vi "day 9 task 1.vi"() -> ()   [LabVIEW 2019]
uses:
  00c26ec4-7482-4959-871a-3b0b3985b684.vi
panel:
  out "Final T pos":cluster{"x":i32, "y":i32}
  out "Final H pos":cluster{"x":i32, "y":i32}
  out "size(s)":i32
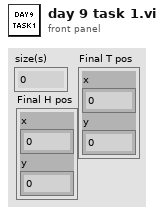
[diagram p1: front panel]
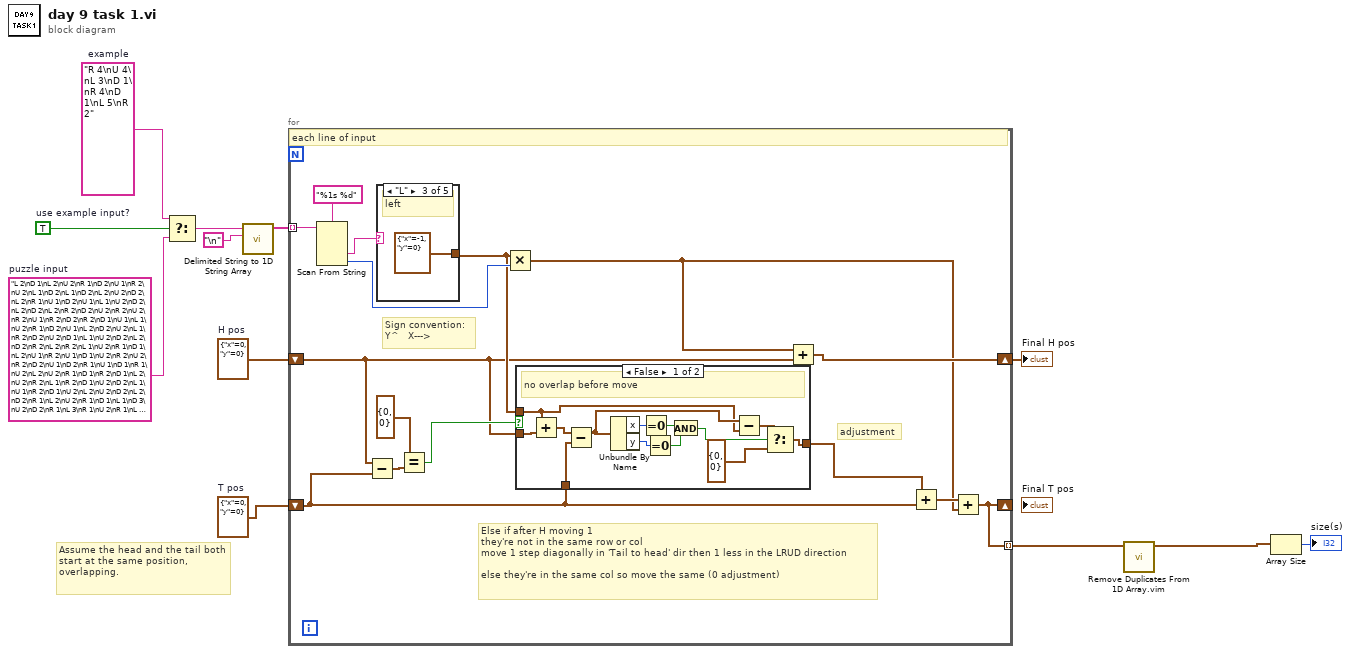
[diagram p0: block diagram]
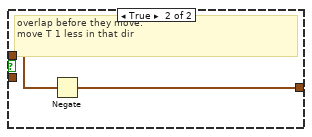
[diagram p2: hidden frame]
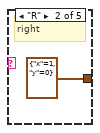
[diagram p4: hidden frame]
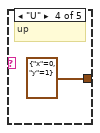
[diagram p5: hidden frame]
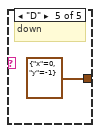
[diagram p6: hidden frame]
diagram:
  w5 = cluster{"x":i32, "y":i32} {"x"=0, "y"=0}  # T pos
  w6 = cluster{"x":i32, "y":i32} {"x"=0, "y"=0}  # H pos
  w10 = "R 4\nU 4\nL 3\nD 1\nR 4\nD 1\nL 5\nR 2"  # example
  w11 = TRUE  # use example input?
  w12 = "L 2\nD 1\nL 2\nU 2\nR 1\nD 2\nU 1\nR 2\nU 2\nL 1\nD 2\nL 1\nD 2\nL 2\nU 2\nD 2\nL 2\nR 1\nU 1\nD 2\nU 1\nL 1\nU 2\nD 2\nL 2\nD 2\nL 2\nR 2\nD 2\nU 2\nR 2\nU 2\nR 2\nU 1\nR 2\nD 2\nR 2\nD 1\nU 1\nL 1\nU 2\nR 1\nD 2\nU 1\nL 2\nD 2\nU 2\nL 1\nR 2\nD 2\nU 2\nD 1\nL 1\nU 2\nD 2\nL 2\nD 2\nR 2\nL 2\nR 2\nL 1\nU 2\nR 1\nD 1\nL 2\nU 1\nR 2\nU 1\nD 1\nU 2\nR 2\nU 2\nR 2\nD 2\nU 1\nD 2\nR 1\nU 1\nD 1\nR 1\nU 2\nL 2\nU 2\nR 1\nD 1\nR 2\nD 1\nL 2\nU 2\nR 2\nL 1\nR 2\nD 1\nU 2\nD 2\nL 1\nU 1\nR 2\nD 1\nU 2\nL 2\nU 2\nD 2\nL 2\nD 2\nR 1\nL 2\nU 2\nR 1\nD 1\nL 1\nD 3\nU 2\nD 2\nR 1\nL 3\nR 1\nU 2\nR 1\nL 2\nU 1\nL 3\nR 2\nU 2\nR 3\nU 3\nL 3\nU 1\nD 1\nR 3\nL 2\nU 1\nR 2\nU 1\nD 3\nU 1\nR 2\nL 2\nD 1\nL 1\nR 3\nU 2\nL 3\nR 2\nD 2\nL 1\nU 2\nR 2\nU 3\nL 1\nR 2\nL 3\nU 3\nL 1\nU 2\nR 2\nU 2\nD 2\nL 2\nU 1\nD 1\nU 2\nD 3\nR 2\nL 2\nU 1\nR 2\nD 3\nU 2\nL 2\nU 1\nR 1\nL 1\nD 1\nL 3\nR 2\nD 2\nL 2\nD 1\nU 3\nD 3\nU 3\nL 3\nR 2\nL 1\nU 2\nR 3\nU 2\nR 2\nU 3\nD 2\nU 1\nL 3\nU 1\nL 1\nD 2\nL 2\nR 1\nL 1\nD 3\nL 2\nD 2\nR 2\nL 3\nR 2\nL 2\nU 1\nL 3\nU 2\nR 2\nD 2\nU 2\nL 1\nD 3\nR 1\nU 3\nD 2\nU 3\nL 1\nD 2\nR 1\nU 3\nR 4\nL 1\nU 4\nR 2\nD 2\nU 3\nD 1\nL 1\nD 4\nL 3\nD 4\nL 3\nD 3\nU 4\nL 2\nD 1\nU 1\nR 4\nD 4\nL 2\nR 3\nU 3\nD 1\nL 3\nD 2\nL 4\nD 4\nR 3\nD 4\nU 4\nR 3\nL 4\nU 1\nL 1\nR 4\nD 2\nR 4\nU 3\nD 2\nR 4\nU 4\nD 1\nU 2\nD 3\nU 2\nL 3\nR 4\nL 1\nU 4\nD 3\nL 4\nR 2\nU 1\nR 1\nD 2\nL 2\nU 2\nL 3\nR 1\nL 2\nD 1\nR 3\nL 4\nU 2\nR 1\nU 1\nR 3\nL 3\nD 2\nU 2\nL 1\nR 1\nL 2\nD 2\nL 1\nR 2\nL 1\nU 1\nR 1\nL 4\nR 3\nU 4\nR 4\nL 2\nR 4\nL 1\nU 2\nR 3\nL 4\nU 1\nR 1\nD 1\nU 3\nL 1\nD 2\nU 2\nD 3\nR 4\nU 1\nR 3\nD 2\nU 1\nD 1\nU 4\nR 2\nD 4\nL 3\nR 4\nU 3\nD 4\nL 3\nU 2\nD 2\nL 4\nD 1\nL 2\nR 2\nU 3\nR 5\nL 3\nU 5\nL 4\nU 3\nD 1\nU 2\nD 5\nL 5\nD 3\nR 3\nD 3\nU 3\nD 5\nU 4\nD 5\nL 5\nR 2\nD 1\nR 5\nU 2\nL 2\nU 5\nL 1\nR 4\nU 5\nR 1\nD 5\nR 3\nU 1\nR 5\nD 5\nL 1\nD 4\nR 5\nL 1\nD 3\nU 2\nD 1\nU 1\nD 4\nL 5\nD 4\nR 1\nL 2\nU 3\nL 1\nU 3\nL 3\nU 4\nL 2\nR 4\nD 5\nU 1\nL 3\nU 5\nR 1\nD 4\nU 3\nL 5\nU 1\nL 3\nD 3\nR 4\nL 5\nU 1\nL 5\nU 2\nD 1\nR 2\nL 2\nD 4\nL 5\nD 2\nR 5\nL 4\nD 1\nR 5\nU 3\nR 2\nD 3\nL 1\nD 1\nL 4\nU 5\nL 2\nD 3\nR 5\nU 2\nL 1\nU 5\nD 4\nU 1\nR 2\nL 1\nU 2\nL 3\nD 1\nU 3\nL 1\nR 5\nU 3\nR 3\nU 2\nR 5\nL 5\nU 1\nL 5\nD 5\nR 1\nU 4\nL 6\nD 4\nU 2\nL 1\nU 5\nL 1\nR 6\nD 3\nU 5\nR 3\nU 5\nD 3\nR 3\nL 2\nU 2\nL 6\nR 3\nU 5\nD 5\nL 6\nR 1\nL 1\nD 5\nU 1\nR 5\nL 4\nR 1\nL 5\nD 1\nL 2\nU 4\nL 5\nU 4\nR 2\nL 1\nD 2\nR 4\nU 5\nD 4\nU 2\nL 3\nR 2\nL 1\nD 3\nU 1\nL 2\nU 6\nL 2\nU 3\nR 2\nD 1\nL 4\nR 5\nL 3\nU 5\nL 6\nR 3\nU 4\nL 2\nR 3\nU 3\nL 1\nD 5\nR 5\nD 5\nU 5\nL 6\nR 5\nL 4\nU 2\nR 5\nU 1\nD 2\nR 2\nD 1\nU 6\nL 5\nD 1\nR 6\nU 5\nR 3\nD 1\nR 4\nD 2\nU 5\nL 5\nR 2\nD 2\nR 1\nU 4\nR 3\nU 4\nL 6\nD 3\nR 4\nL 4\nU 5\nD 1\nU 1\nD 5\nU 4\nL 5\nD 1\nR 1\nU 5\nD 7\nR 5\nD 2\nR 2\nD 7\nL 1\nR 2\nD 2\nR 7\nU 4\nD 3\nU 3\nD 3\nL 4\nD 2\nR 6\nL 7\nD 6\nU 4\nD 1\nL 4\nU 3\nD 1\nU 1\nL 6\nD 4\nL 7\nU 6\nR 4\nL 7\nU 2\nD 5\nL 7\nU 3\nR 3\nU 6\nR 7\nU 4\nR 4\nL 4\nU 6\nR 6\nD 7\nU 4\nD 5\nL 4\nU 7\nR 7\nD 3\nL 5\nU 7\nD 3\nU 1\nD 7\nR 7\nL 4\nU 7\nD 1\nR 3\nD 3\nU 4\nR 2\nU 4\nR 4\nU 7\nR 4\nL 2\nU 4\nR 7\nL 6\nU 1\nD 2\nU 3\nD 1\nL 6\nD 5\nL 7\nR 6\nD 6\nL 4\nD 4\nU 3\nD 3\nL 7\nR 7\nL 7\nD 6\nU 5\nD 7\nU 7\nD 4\nU 7\nL 6\nU 3\nD 3\nR 3\nD 4\nL 2\nU 2\nR 4\nD 5\nR 7\nU 7\nL 2\nU 1\nD 4\nU 3\nL 4\nU 6\nD 4\nL 4\nU 6\nD 5\nL 1\nR 4\nL 2\nD 6\nR 4\nD 3\nR 3\nL 1\nD 2\nU 3\nL 1\nU 7\nL 3\nR 5\nU 1\nL 4\nD 8\nL 7\nD 8\nL 4\nU 6\nR 2\nD 4\nR 3\nD 3\nR 6\nL 8\nR 6\nD 4\nL 5\nR 5\nD 3\nU 6\nD 5\nU 3\nL 1\nD 4\nU 2\nR 5\nD 8\nL 3\nD 2\nU 8\nL 2\nD 6\nL 6\nD 2\nR 8\nL 3\nD 8\nU 5\nL 1\nR 1\nD 3\nL 5\nR 7\nU 4\nD 1\nL 2\nD 2\nL 5\nD 7\nR 7\nU 5\nL 5\nD 6\nL 1\nU 3\nL 4\nR 6\nD 7\nU 1\nR 1\nL 8\nU 3\nD 4\nR 2\nD 8\nL 1\nR 8\nU 7\nL 6\nU 4\nD 4\nL 2\nD 8\nU 8\nR 4\nU 3\nD 7\nR 6\nD 8\nR 5\nL 4\nD 4\nL 8\nD 3\nR 4\nL 6\nU 8\nD 1\nL 3\nR 7\nL 4\nU 3\nD 2\nU 4\nR 2\nD 1\nU 5\nL 7\nU 3\nL 8\nU 1\nL 4\nR 4\nU 1\nR 2\nL 4\nU 8\nD 7\nL 8\nD 4\nU 3\nD 5\nU 2\nD 2\nR 1\nU 6\nL 3\nR 8\nU 2\nR 2\nD 7\nL 3\nU 3\nR 8\nU 4\nR 7\nU 5\nR 7\nD 4\nR 4\nD 7\nU 5\nL 2\nD 2\nL 3\nU 2\nD 2\nL 6\nR 6\nL 5\nU 9\nD 3\nL 4\nU 3\nL 7\nD 6\nL 6\nU 7\nR 8\nU 8\nL 9\nD 7\nL 9\nD 1\nL 1\nR 7\nU 7\nL 5\nD 9\nR 8\nL 1\nR 5\nL 3\nD 3\nU 1\nR 8\nU 6\nD 3\nR 5\nU 4\nL 1\nR 3\nL 1\nU 7\nD 3\nR 3\nD 8\nR 5\nU 2\nR 5\nD 1\nL 5\nD 5\nR 6\nL 1\nD 9\nL 2\nD 9\nU 4\nL 1\nD 8\nL 2\nU 2\nD 7\nU 9\nL 8\nD 1\nR 2\nL 3\nD 4\nL 6\nU 5\nD 5\nU 1\nL 5\nU 7\nD 7\nL 9\nD 8\nR 8\nU 1\nD 9\nL 8\nU 9\nD 2\nR 6\nL 3\nU 6\nR 3\nU 5\nD 8\nL 5\nD 9\nU 5\nR 4\nU 5\nR 1\nL 5\nU 4\nL 4\nD 1\nL 1\nD 7\nR 7\nU 2\nL 5\nR 9\nU 6\nD 2\nU 6\nR 1\nD 8\nU 6\nD 3\nU 10\nD 5\nL 6\nR 6\nL 5\nD 7\nU 3\nL 4\nD 3\nR 10\nU 8\nD 3\nL 1\nR 9\nL 2\nR 9\nU 10\nD 3\nU 6\nR 8\nD 4\nR 7\nL 1\nU 8\nD 7\nR 2\nU 8\nD 8\nL 7\nU 6\nR 4\nD 4\nR 1\nU 4\nR 2\nL 5\nD 8\nU 4\nL 8\nU 1\nD 1\nL 6\nU 10\nR 10\nL 9\nU 6\nL 2\nU 2\nL 1\nU 1\nL 6\nD 4\nU 2\nD 6\nU 4\nD 10\nR 8\nD 8\nR 8\nD 2\nU 6\nL 9\nD 2\nL 4\nD 3\nL 4\nR 3\nU 2\nD 1\nU 1\nR 1\nD 7\nU 3\nR 10\nD 1\nU 6\nR 2\nD 1\nR 11\nD 1\nR 7\nU 4\nD 8\nU 7\nR 11\nL 10\nR 7\nL 3\nD 1\nU 2\nL 9\nR 5\nL 6\nR 6\nU 2\nR 3\nU 8\nD 6\nU 7\nL 6\nD 11\nL 10\nD 3\nR 3\nU 11\nD 7\nU 2\nR 1\nL 6\nR 2\nL 2\nD 3\nL 8\nR 6\nD 10\nU 6\nD 11\nL 7\nR 11\nD 2\nL 9\nU 7\nD 5\nU 5\nD 11\nL 4\nR 8\nD 9\nL 4\nU 1\nR 6\nD 11\nU 6\nL 5\nU 3\nL 11\nD 8\nU 2\nD 9\nR 2\nL 10\nU 8\nD 7\nU 3\nL 7\nD 10\nL 7\nD 10\nR 1\nD 10\nL 7\nU 3\nL 1\nR 9\nD 5\nL 11\nR 3\nL 9\nR 8\nD 2\nU 5\nL 4\nD 2\nU 7\nR 9\nU 9\nL 2\nD 1\nR 6\nL 5\nD 8\nU 8\nR 6\nU 3\nL 7\nU 4\nR 7\nL 1\nD 7\nR 2\nU 10\nD 3\nU 4\nR 8\nD 5\nL 8\nD 5\nU 8\nR 6\nU 2\nL 8\nU 7\nL 12\nD 11\nL 8\nD 12\nR 10\nL 10\nU 7\nD 2\nR 6\nL 11\nU 4\nD 8\nU 11\nL 1\nD 12\nL 3\nR 10\nD 2\nR 4\nL 1\nD 2\nR 2\nL 12\nU 3\nL 10\nU 4\nD 10\nU 8\nL 5\nR 5\nL 12\nU 1\nD 10\nU 2\nD 12\nU 12\nR 2\nU 1\nR 4\nD 8\nL 9\nR 7\nL 5\nD 5\nU 5\nL 7\nU 2\nL 7\nU 6\nL 12\nU 11\nR 10\nU 3\nL 4\nD 6\nR 11\nU 3\nR 5\nL 2\nU 9\nR 2\nL 10\nD 3\nU 12\nR 9\nD 2\nU 12\nL 1\nU 9\nD 9\nL 2\nD 4\nR 11\nD 2\nL 2\nU 12\nR 10\nD 6\nU 11\nR 9\nD 12\nL 2\nU 11\nL 5\nU 6\nR 7\nU 9\nL 10\nR 1\nL 3\nR 3\nD 2\nR 5\nL 12\nR 1\nU 3\nD 1\nL 3\nU 5\nD 9\nL 10\nU 9\nD 11\nL 12\nU 7\nR 12\nL 3\nD 2\nR 10\nU 13\nR 6\nL 5\nU 12\nL 2\nR 13\nU 8\nD 3\nR 8\nL 3\nR 3\nD 9\nR 6\nD 10\nR 2\nU 12\nR 1\nD 2\nR 12\nD 7\nU 3\nL 13\nR 11\nD 4\nU 9\nL 12\nU 3\nL 7\nD 2\nL 12\nD 12\nR 10\nD 11\nU 7\nR 4\nU 10\nR 11\nL 11\nR 7\nD 13\nU 11\nR 11\nU 3\nL 6\nU 9\nD 1\nU 3\nD 13\nR 10\nU 3\nR 3\nD 7\nU 6\nL 11\nR 10\nD 9\nR 12\nD 5\nR 7\nD 3\nR 5\nL 1\nR 10\nL 8\nD 12\nR 2\nU 9\nR 13\nU 13\nR 12\nL 8\nD 13\nR 1\nL 6\nU 10\nD 2\nU 7\nL 6\nU 6\nR 7\nU 12\nR 10\nU 12\nL 5\nD 4\nL 8\nU 12\nL 13\nD 6\nR 1\nD 2\nL 10\nU 13\nR 12\nD 4\nL 8\nR 11\nD 5\nU 11\nD 7\nL 1\nU 12\nL 6\nU 12\nD 7\nL 8\nR 13\nD 12\nR 11\nD 2\nU 14\nL 5\nD 2\nL 6\nU 14\nL 1\nU 2\nR 12\nL 9\nU 14\nD 2\nU 5\nD 3\nU 11\nR 7\nU 5\nR 13\nD 5\nL 2\nR 12\nU 6\nD 1\nU 14\nD 3\nL 13\nU 2\nD 2\nU 1\nD 12\nU 12\nD 4\nU 2\nD 2\nR 8\nU 3\nD 13\nR 2\nD 6\nU 11\nD 12\nL 3\nU 7\nD 14\nL 4\nU 11\nL 4\nD 2\nR 13\nL 6\nU 9\nR 14\nU 10\nD 11\nL 12\nR 4\nD 9\nR 11\nD 8\nR 7\nD 12\nR 7\nU 4\nL 8\nD 7\nR 9\nU 7\nR 13\nU 3\nR 11\nD 7\nU 3\nR 9\nL 8\nU 2\nD 5\nU 8\nD 1\nL 8\nU 12\nR 13\nL 7\nR 8\nL 10\nR 2\nD 13\nL 12\nR 2\nL 7\nR 9\nU 7\nD 8\nL 10\nD 12\nU 14\nR 5\nD 11\nL 12\nU 4\nL 1\nD 5\nU 6\nD 9\nU 8\nR 8\nD 11\nR 6\nU 5\nR 1\nL 15\nD 5\nU 1\nR 6\nD 8\nR 15\nU 15\nR 3\nD 14\nL 1\nD 2\nL 13\nR 13\nU 5\nL 6\nD 10\nR 7\nU 4\nD 15\nR 14\nD 12\nU 4\nD 12\nU 12\nL 12\nR 8\nL 15\nD 1\nR 6\nU 5\nD 7\nR 8\nU 7\nD 6\nU 1\nD 1\nL 2\nR 3\nD 13\nU 4\nD 4\nU 6\nL 13\nD 10\nR 14\nL 10\nD 15\nU 12\nR 10\nD 13\nL 1\nR 13\nD 10\nU 2\nR 5\nD 3\nU 13\nD 1\nR 15\nU 4\nL 8\nD 6\nL 13\nR 4\nL 11\nD 15\nU 11\nL 13\nD 6\nL 15\nU 9\nL 1\nR 11\nU 14\nR 6\nL 12\nR 5\nU 5\nL 11\nD 13\nU 3\nL 4\nR 1\nD 11\nL 8\nD 9\nR 12\nD 14\nU 15\nD 14\nU 14\nL 14\nU 4\nL 13\nD 8\nU 13\nR 7\nL 11\nD 15\nL 5\nU 7\nR 10\nD 13\nR 15\nD 2\nR 2\nL 10\nR 4\nU 7\nD 15\nL 6\nD 9\nL 16\nR 10\nU 3\nR 6\nL 8\nU 15\nR 4\nD 1\nU 8\nL 14\nR 6\nU 8\nL 10\nD 4\nU 9\nR 4\nD 1\nU 4\nL 2\nR 16\nL 6\nD 16\nU 14\nR 10\nL 14\nU 3\nR 7\nU 6\nR 13\nL 5\nR 15\nL 7\nR 3\nD 16\nL 11\nU 12\nL 11\nD 8\nR 7\nL 11\nR 5\nU 8\nR 2\nU 10\nR 11\nU 1\nD 14\nU 14\nR 4\nL 6\nD 4\nU 16\nD 2\nR 12\nL 6\nU 7\nL 7\nD 8\nR 4\nD 8\nU 11\nL 13\nU 9\nD 8\nL 8\nU 16\nD 3\nL 1\nR 13\nU 2\nL 12\nR 2\nL 3\nD 11\nR 4\nL 12\nR 12\nU 4\nD 8\nL 12\nU 16\nL 9\nR 5\nU 13\nL 1\nR 10\nL 15\nU 2\nR 8\nL 8\nD 11\nR 7\nL 7\nR 2\nL 13\nD 11\nL 11\nD 7\nL 8\nU 11\nR 7\nL 15\nD 5\nL 13\nR 8\nD 4\nR 6\nL 1\nU 10\nL 17\nU 16\nR 6\nD 17\nU 14\nL 13\nD 3\nU 11\nR 10\nD 3\nL 15\nU 13\nR 7\nL 12\nU 3\nL 7\nR 13\nL 10\nR 13\nL 10\nD 1\nR 11\nL 12\nU 6\nR 2\nL 4\nR 11\nU 15\nD 6\nL 15\nR 7\nU 16\nD 9\nL 12\nD 14\nL 5\nD 15\nL 17\nR 7\nU 17\nL 10\nD 7\nL 2\nD 1\nU 4\nD 17\nU 17\nD 9\nL 14\nD 16\nL 2\nD 8\nL 5\nD 8\nR 6\nL 15\nR 17\nD 14\nU 17\nL 17\nU 12\nR 10\nL 12\nU 16\nR 10\nD 5\nR 2\nU 11\nR 6\nL 2\nR 2\nD 17\nU 17\nD 12\nU 5\nL 14\nU 2\nR 2\nD 3\nU 4\nR 5\nU 17\nL 9\nU 4\nR 2\nL 5\nU 8\nL 2\nD 5\nR 14\nU 15\nR 14\nD 3\nU 16\nL 3\nD 6\nU 3\nL 2\nR 3\nL 1\nR 6\nL 14\nU 10\nL 13\nR 8\nU 3\nD 7\nU 9\nD 2\nL 14\nD 5\nR 7\nD 8\nL 18\nR 13\nU 14\nD 6\nR 10\nL 10\nU 2\nL 11\nR 12\nU 6\nR 16\nL 10\nU 7\nR 12\nL 15\nD 2\nU 16\nL 4\nD 2\nL 1\nR 8\nD 7\nL 11\nR 4\nD 13\nU 13\nR 1\nD 15\nL 12\nR 5\nD 10\nU 8\nR 14\nL 10\nU 9\nR 7\nU 13\nL 5\nU 9\nL 15\nR 4\nD 13\nR 12\nD 5\nR 18\nL 3\nD 13\nR 17\nD 9\nL 8\nD 3\nL 5\nD 8\nU 10\nD 8\nL 2\nU 10\nR 6\nD 13\nL 17\nR 17\nD 16\nR 14\nL 6\nU 17\nR 9\nD 11\nL 7\nU 16\nR 16\nL 1\nR 17\nD 9\nL 6\nD 16\nR 12\nL 7\nU 5\nD 14\nR 8\nU 12\nL 12\nR 8\nU 17\nL 13\nD 17\nL 15\nR 7\nU 11\nL 10\nR 8\nU 14\nR 6\nU 11\nD 17\nU 13\nL 12\nU 11\nL 16\nD 13\nU 11\nL 2\nR 11\nL 13\nU 12\nR 15\nU 17\nL 10\nU 17\nD 2\nR 1\nL 10\nR 10\nU 14\nL 12\nU 8\nR 4\nL 12\nU 13\nL 2\nR 9\nD 14\nU 17\nL 16\nD 9\nR 3\nL 17\nU 8\nR 16\nD 11\nL 1\nU 15\nL 19\nR 8\nD 11\nR 14\nD 19\nR 12\nU 3\nL 9\nU 2\nL 6\nD 6\nU 16\nD 4\nL 1\nD 10\nR 8\nU 17\nD 2\nR 6\nD 19\nU 6\nR 9\nU 17\nD 7\nL 15\nD 13\nL 17\nU 1\nR 17\nD 3\nL 15\nU 16\nD 13\nR 13\nD 14\nL 12\nD 4\nL 16\nU 15\nR 8\nU 19\nD 15\nL 5\nR 15\nL 19\nU 6\nD 6\nU 10\nL 1\nR 19\nL 1\nR 6\nL 1\nU 17\nR 10\nU 4\nD 5\nR 6\nU 3\nR 12\nU 13\nD 7\nR 15\nU 5\nR 2\nU 10\nL 13\nU 3\nD 5\nR 19\nU 9\nD 5\nL 3\nD 17\nL 16\nD 7\nL 16\nR 11\nD 3\nU 1\nR 2\nD 2\nL 4\nR 4\nU 17\nD 4\nL 10\nU 11\nD 13"  # puzzle input
  # "Assume the head and the tail both start at the same position, overlapping."
  n1 = Select(t=w10, s=w11, f=w12) -> (s? t:f=w9:string)
  n2 = call <vilib>:"Delimited String to 1D String Array.vi"("delimiter"="\n", "delimited string"=w9) -> ("string array"=w7:string[])  [unwired: 9 in]
  n3 = for {
    tunnel: w7 -> [w27] mode=indexing
    shift-right: [w23] -> w2
    shift-left: w6 -> [w15]
    shift-right: [w13] -> _
    shift-left: w5 -> [w14]
    tunnel: [w13] -> w1 mode=indexing
    # "adjustment"
    # "Else if after H moving 1\nthey're not in the same row or col\nmove 1 step diagonally in 'Tail to head' dir then 1 less in the LRUD direction\n\nelse they're in the same col so move the same (0 adjustment)"
    # "Sign convention:\nY^   X--->"
    # "each line of input"
    n4 = Scan From String(format string="%1s %d", input string=w27) -> (output 1=w25:string, output 2=w24:i32)  [unwired: 4 in, 3 out]
    n5 = Subtract(x=w15, y=w14) -> (x-y=w22:cluster{"x":i32, "y":i32})
    n6 = case shown="\"L\"" w25 {
      tunnel: [_ cluster{"x":i32, "y":i32} {"x"=1, "y"=0} ("movement") cluster{"x":i32, "y":i32} {"x"=-1, "y"=0} ("movement") cluster{"x":i32, "y":i32} {"x"=0, "y"=1} ("movement") cluster{"x":i32, "y":i32} {"x"=0, "y"=-1} ("movement")] -> w16
      frame Default {
      }
      frame "R" {
        # "right"
      }
      frame "L" {
        # "left"
      }
      frame "U" {
        # "up"
      }
      frame "D" {
        # "down"
      }
    }
    n7 = Equal?(x=cluster{"x":i32, "y":i32} {"x"=0, "y"=0}, y=w22) -> (x = y?=w18:bool)
    n8 = Multiply(x=w16, y=w24) -> (x*y=w19:cluster{"x":i32, "y":i32})
    n9 = case shown="False" w18 {
      tunnel: [w33 w41] -> w17
      tunnel: w16 -> [w29 w42]
      tunnel: w15 -> [w38 _]
      tunnel: w14 -> [w36 _]
      frame False {
        # "no overlap before move"
        n10 = Add(x=w29, y=w38) -> (x+y=w37:cluster{"x":i32, "y":i32})
        n11 = Subtract(x=w37, y=w36) -> (x-y=w30:cluster{"x":i32, "y":i32})
        n12 = Unbundle By Name(w30) -> ("x"=w35:i32, "y"=w34:i32)
        n13 = Equal To 0?(x=w35) -> (x = 0?=w39:bool)
        n14 = Equal To 0?(x=w34) -> (x = 0?=w40:bool)
        n15 = And(x=w39, y=w40) -> (x .and. y?=w32:bool)
        n16 = Subtract(x=w30, y=w29) -> (x-y=w28:cluster{"x":i32, "y":i32})
        n17 = Select(t=w28, s=w32, f=cluster{"x":i32, "y":i32} {"x"=0, "y"=0}) -> (s? t:f=w33:cluster{"x":i32, "y":i32})
      }
      frame True {
        # "overlap before they move:\nmove T 1 less in that dir"
        n18 = Negate(x=w42) -> (-x=w41:cluster{"x":i32, "y":i32})
      }
    }
    n19 = Add(x=w19, y=w15) -> (x+y=w23:cluster{"x":i32, "y":i32})
    n20 = Add(x=w17, y=w14) -> (x+y=w20:cluster{"x":i32, "y":i32})
    n21 = Add(x=w20, y=w19) -> (x+y=w13:cluster{"x":i32, "y":i32})
  }
  "Final H pos" <- w2
  n22 = call "Remove Duplicates From 1D Array.vim"("array"=w1) -> ("array with duplicates removed"=w4:cluster{"x":i32, "y":i32}[])  [unwired: 10 in]
  n23 = Array Size(array=w4) -> (size(s)=→"size(s)":i32)
